vi "EOL AP Check Data.vi"(5 "Raw Rollo AP Data":string, 7 "Raw Glass AP Data":string, 8 "error in":errorcluster, 9 "Error Table":string[][](array[string]), 10 "Database AP Data":dbl[](array[numeric])) -> (0 "error out":errorcluster, 1 "Error Table Out":string[][](array[string]), 3 "Pass? Out":bool)   [LabVIEW 2018]
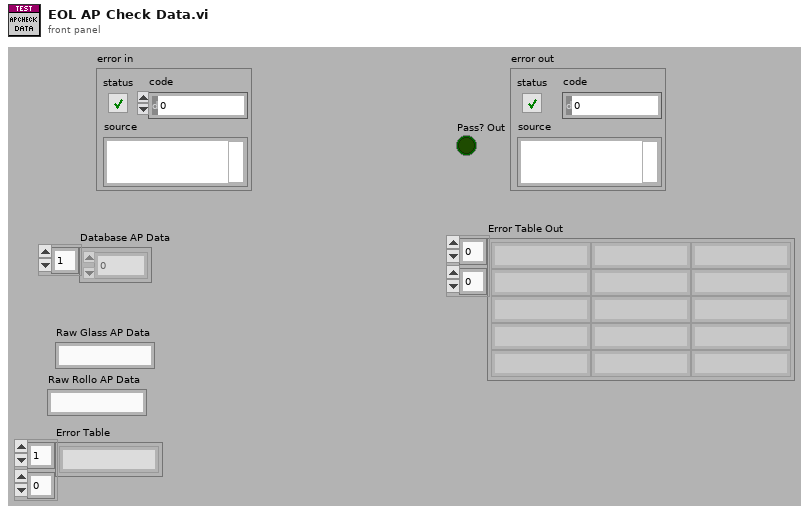
[diagram p1: front panel]
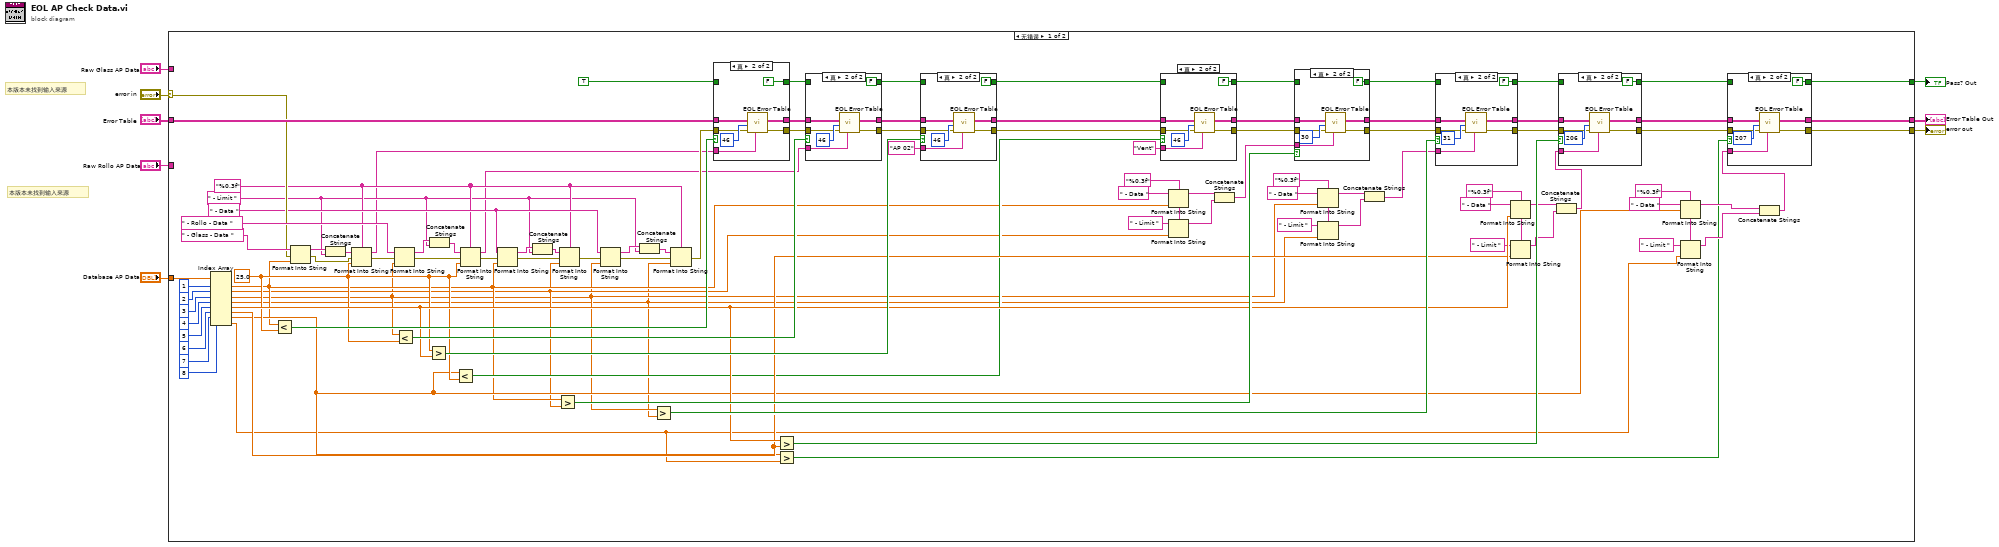
[diagram p0: block diagram]
diagram:
  # "本版本未找到输入来源"
  # "本版本未找到输入来源"
  n1 = case shown="无错误" "error in" {
    selector: "error in" -> [w76 w192]
    tunnel: "Error Table" -> [w100 w191]
    tunnel: "Raw Glass AP Data" -> [_ _]
    tunnel: [w33 _] -> w6
    tunnel: [w37 w191] -> w5
    tunnel: "Raw Rollo AP Data" -> [_ _]
    tunnel: "Database AP Data" -> [w87 _]
    tunnel: [w35 w192] -> w2
    frame No Error {
      w14 = "%0.3f" ("format string")
      w25 = "%0.3f" ("format string")
      w41 = "%0.3f" ("format string")
      w55 = "%0.3f" ("format string")
      w74 = "%0.3f" ("format string")
      w73 = " - Limit " ("initial string")
      w75 = " - Data " ("initial string")
      w50 = 25.0 ("y")
      n2 = Index Array(array=w87, index #1=1 ("index"), index #2=2 ("index"), index #3=3 ("index"), index #4=4 ("index"), index #5=5 ("index"), index #6=6 ("index"), index #7=7 ("index"), index #8=8 ("index")) -> (element #1=w21:dbl, element #2=w20:dbl, element #3=w12:dbl, element #4=w11:dbl, element #5=w60:dbl, element #6=w57:dbl, element #7=w28:dbl, element #8=w27:dbl)
      n3 = Less?(x=w21, y=w50) -> (x < y?=w110:bool)
      n4 = Format Into String(initial string=" - Glass - Data ", error in=w76, w21) -> (resulting string=w108:string, error out=w86:errorcluster)  [unwired: 1 in]
      n5 = Concatenate Strings(w108, w73) -> (w109:string)
      n6 = Format Into String(format string=w74, initial string=w109, error in=w86, w50) -> (resulting string=w18:string, error out=w85:errorcluster)
      n7 = Format Into String(initial string=" - Rollo - Data ", error in=w85, w12) -> (resulting string=w107:string, error out=w84:errorcluster)  [unwired: 1 in]
      n8 = Less?(x=w12, y=w50) -> (x < y?=w104:bool)
      n9 = Greater?(x=w50, y=w60) -> (0:w69:bool)
      n10 = Concatenate Strings(w107, w73) -> (w106:string)
      n11 = Less?(x=w28, y=w50) -> (x < y?=w42:bool)
      n12 = Format Into String(format string=w74, initial string=w106, error in=w84, w50) -> (resulting string=w9:string, error out=w83:errorcluster)
      n13 = Format Into String(initial string=w75, error in=w83, w21) -> (resulting string=w97:string, error out=w82:errorcluster)  [unwired: 1 in]
      n14 = Concatenate Strings(w97, w73) -> (w98:string)
      n15 = Greater?(x=w21, y=w20) -> (0:w99:bool)
      n16 = Format Into String(format string=w74, initial string=w98, error in=w82, w20) -> (error out=w81:errorcluster)  [unwired: 1 out]
      n17 = Format Into String(initial string=w75, error in=w81, w12) -> (resulting string=w96:string, error out=w80:errorcluster)  [unwired: 1 in]
      n18 = Concatenate Strings(w96, w73) -> (w95:string)
      n19 = Greater?(x=w12, y=w11) -> (0:w93:bool)
      n20 = Format Into String(format string=w74, initial string=w95, error in=w80, w11) -> (error out=w79:errorcluster)  [unwired: 1 out]
      n21 = case shown="真" w110 {
        tunnel: w100 -> [w183 w190]
        tunnel: [w183 w186] -> w105
        tunnel: w18 -> [_ w188]
        tunnel: TRUE ("Pass?") -> [w182 _]
        tunnel: [w182 FALSE ("Pass?")] -> w103
        tunnel: w79 -> [w181 w185]
        tunnel: [w181 w184] -> w78
        frame False {
        }
        frame True {
          n22 = call "EOL Error Table.vi"("Error Description"=w188, "error in"=w185, "Error No."=u16 46, "Error Table In"=w190) -> ("error out"=w184:errorcluster, "Error Table Out"=w186:string[][])  [unwired: 6 in]
        }
      }
      n23 = Greater?(x=w60, y=w57) -> (0:w61:bool)
      n24 = Greater?(x=w28, y=w27) -> (0:w29:bool)
      n25 = case shown="真" w104 {
        tunnel: w105 -> [w173 w180]
        tunnel: [w173 w176] -> w68
        tunnel: w9 -> [_ w177]
        tunnel: w103 -> [w172 _]
        tunnel: [w172 FALSE ("Pass?")] -> w65
        tunnel: w78 -> [w171 w175]
        tunnel: [w171 w174] -> w67
        frame False {
        }
        frame True {
          n26 = call "EOL Error Table.vi"("Error Description"=w177, "error in"=w175, "Error No."=u16 46, "Error Table In"=w180) -> ("error out"=w174:errorcluster, "Error Table Out"=w176:string[][])  [unwired: 6 in]
        }
      }
      n27 = case shown="真" w69 {
        tunnel: w68 -> [w143 w150]
        tunnel: [w143 w146] -> w46
        tunnel: "AP 02" ("Raw Rollo AP Data") -> [_ w147]
        tunnel: w65 -> [w142 _]
        tunnel: [w142 FALSE ("Pass?")] -> w48
        tunnel: w67 -> [w141 w145]
        tunnel: [w141 w144] -> w44
        frame False {
        }
        frame True {
          n28 = call "EOL Error Table.vi"("Error Description"=w147, "error in"=w145, "Error No."=u16 46, "Error Table In"=w150) -> ("error out"=w144:errorcluster, "Error Table Out"=w146:string[][])  [unwired: 6 in]
        }
      }
      n29 = case shown="真" w42 {
        tunnel: w46 -> [w123 w130]
        tunnel: [w123 w126] -> w45
        tunnel: "Vent" ("Raw Rollo AP Data") -> [_ w127]
        tunnel: w48 -> [w122 _]
        tunnel: [w122 FALSE ("Pass?")] -> w47
        tunnel: w44 -> [w121 w125]
        tunnel: [w121 w124] -> w43
        frame False {
        }
        frame True {
          n30 = call "EOL Error Table.vi"("Error Description"=w127, "error in"=w125, "Error No."=u16 46, "Error Table In"=w130) -> ("error out"=w124:errorcluster, "Error Table Out"=w126:string[][])  [unwired: 6 in]
        }
      }
      n31 = Format Into String(format string=w25, initial string=" - Data ", w21) -> (resulting string=w23:string)  [unwired: 1 in, 1 out]
      n32 = Format Into String(format string=w25, initial string=" - Limit ", w20) -> (resulting string=w26:string)  [unwired: 1 in, 1 out]
      n33 = Concatenate Strings(w23, w26) -> (w19:string)
      n34 = case shown="真" w99 {
        tunnel: w45 -> [w163 w170]
        tunnel: [w163 w166] -> w94
        tunnel: w19 -> [_ w167]
        tunnel: w47 -> [w162 _]
        tunnel: [w162 FALSE ("Pass?")] -> w92
        tunnel: w43 -> [w161 w165]
        tunnel: [w161 w164] -> w77
        frame False {
        }
        frame True {
          n35 = call "EOL Error Table.vi"("Error Description"=w167, "error in"=w165, "Error No."=u16 30, "Error Table In"=w170) -> ("error out"=w164:errorcluster, "Error Table Out"=w166:string[][])  [unwired: 6 in]
        }
      }
      n36 = Format Into String(format string=w14, initial string=" - Data ", w12) -> (resulting string=w16:string)  [unwired: 1 in, 1 out]
      n37 = Format Into String(format string=w14, initial string=" - Limit ", w11) -> (resulting string=w13:string)  [unwired: 1 in, 1 out]
      n38 = Concatenate Strings(w16, w13) -> (w10:string)
      n39 = case shown="真" w93 {
        tunnel: w94 -> [w153 w160]
        tunnel: [w153 w157] -> w64
        tunnel: w10 -> [_ w156]
        tunnel: w92 -> [w152 _]
        tunnel: [w152 FALSE ("Pass?")] -> w62
        tunnel: w77 -> [w151 w155]
        tunnel: [w151 w154] -> w63
        frame False {
        }
        frame True {
          n40 = call "EOL Error Table.vi"("Error Description"=w156, "error in"=w155, "Error No."=u16 31, "Error Table In"=w160) -> ("error out"=w154:errorcluster, "Error Table Out"=w157:string[][])  [unwired: 6 in]
        }
      }
      n41 = Format Into String(format string=w55, initial string=" - Data ", w60) -> (resulting string=w58:string)  [unwired: 1 in, 1 out]
      n42 = Format Into String(format string=w55, initial string=" - Limit ", w57) -> (resulting string=w54:string)  [unwired: 1 in, 1 out]
      n43 = Concatenate Strings(w58, w54) -> (w53:string)
      n44 = case shown="真" w61 {
        tunnel: w64 -> [w133 w140]
        tunnel: [w133 w137] -> w38
        tunnel: w53 -> [_ w136]
        tunnel: w62 -> [w132 _]
        tunnel: [w132 FALSE ("Pass?")] -> w34
        tunnel: w63 -> [w131 w135]
        tunnel: [w131 w134] -> w36
        frame False {
        }
        frame True {
          n45 = call "EOL Error Table.vi"("Error Description"=w136, "error in"=w135, "Error No."=u16 206, "Error Table In"=w140) -> ("error out"=w134:errorcluster, "Error Table Out"=w137:string[][])  [unwired: 6 in]
        }
      }
      n46 = Format Into String(format string=w41, initial string=" - Data ", w28) -> (resulting string=w32:string)  [unwired: 1 in, 1 out]
      n47 = Format Into String(format string=w41, initial string=" - Limit ", w27) -> (resulting string=w31:string)  [unwired: 1 in, 1 out]
      n48 = Concatenate Strings(w32, w31) -> (w30:string)
      n49 = case shown="真" w29 {
        tunnel: w38 -> [w113 w120]
        tunnel: [w113 w117] -> w37
        tunnel: w30 -> [_ w116]
        tunnel: w34 -> [w112 _]
        tunnel: [w112 FALSE ("Pass?")] -> w33
        tunnel: w36 -> [w111 w115]
        tunnel: [w111 w114] -> w35
        frame False {
        }
        frame True {
          n50 = call "EOL Error Table.vi"("Error Description"=w116, "error in"=w115, "Error No."=u16 207, "Error Table In"=w120) -> ("error out"=w114:errorcluster, "Error Table Out"=w117:string[][])  [unwired: 6 in]
        }
      }
    }
    frame Error {
    }
  }
  "Pass? Out" <- w6
  "Error Table Out" <- w5
  "error out" <- w2
